vi "DAQ IV.vi"() -> ()   [LabVIEW 2024]
uses:
  global.vi
panel:
  in  "base path":path=path "C:/Users/gyue/Desktop/20211027"
  out "Voltage Applied":dbl=-2.0
  in  "Tab Control":enum32{"Curve Control", "Setup"}(tab)
  in  "Voltage Offset":dbl caption="Delay Time (s)" format="%#_4f"
  in  "End Current uA":dbl=2.0
  in  "Start Current uA":dbl=-2.0
  in  "Step uA":dbl=0.05
  in  "Delay Time s":dbl caption="Delay Time (s)"
  in  "True is round":bool=TRUE
  in  "Current scale":dbl=1.0 caption="Delay Time (s)" format="%#_5f"
  in  "Voltage scale":dbl=0.0001 caption="Delay Time (s)" format="%#_4f"
  in  "Wire Resistance":dbl caption="Delay Time (s)" format="%#_6f"
  in  "AO channel":tag="Dev1/ao0"
  in  "AI channel":tag="Dev1/ai1"
  in  "samples per read":i32=1000
  in  "device in":tag="Dev1"
  in  "stop 2":bool
  in  "stop":bool
  out "Cursor measured \nResistance Ohm":dbl=20.21557814005861
  in  "error in":T1
  out "Current Applied":dbl=-2.0
  out "Voltage":dbl=-2.7920312698574086e-05 format="%^#_4g"
  out "IV curve":cluster{"Y":dbl[], "Y":dbl[]}[](graph)=[{"Y"=[-2.0, -1.95, -1.9, -1.85, -1.8, -1.75, -1.7, -1.65, -1.6, -1.55, -1.5, -1.45, -1.4, -1.35, -1.2999999999999998, -1.25, -1.2, -1.15, -1.1, -1.0499999999999998, -1.0, -0.95, -0.8999999999999999, -0.8499999999999999, -0.7999999999999998, -0.75, -0.7, -0.6499999999999999, -0.5999999999999999, -0.5499999999999998, -0.5, -0.44999999999999996, -0.3999999999999999, -0.34999999999999987, -0.2999999999999998, -0.25, -0.19999999999999996, -0.1499999999999999, -0.09999999999999987, -0.04999999999999982, 0.0, 0.050000000000000266, 0.10000000000000009, 0.1499999999999999, 0.20000000000000018, 0.25, 0.30000000000000027, 0.3500000000000001, 0.40000000000000036, 0.4500000000000002, 0.5, 0.5500000000000003, 0.6000000000000001, 0.6500000000000004, 0.7000000000000002, 0.75, 0.8000000000000003, 0.8500000000000001, 0.9000000000000004, 0.9500000000000002, 1.0, 1.0500000000000003, 1.1, 1.1500000000000004, 1.2000000000000002, 1.25, 1.3000000000000003, 1.35, 1.4000000000000004, 1.4500000000000002, 1.5, 1.5500000000000003, 1.6, 1.6500000000000004, 1.7000000000000002, 1.75, 1.8000000000000003, 1.85, 1.9000000000000004, 1.9500000000000002, 2.0, 1.9500000000000002, 1.8999999999999995, 1.8499999999999996, 1.7999999999999998, 1.75, 1.7000000000000002, 1.6499999999999995, 1.5999999999999996, 1.5499999999999998, 1.5, 1.4500000000000002, 1.3999999999999995, 1.3499999999999996, 1.2999999999999998, 1.25, 1.1999999999999993, 1.1499999999999995, 1.0999999999999996, 1.0499999999999998, 1.0, 0.9499999999999993, 0.8999999999999995, 0.8499999999999996, 0.7999999999999998, 0.75, 0.6999999999999993, 0.6499999999999995, 0.5999999999999996, 0.5499999999999998, 0.5, 0.4499999999999993, 0.39999999999999947, 0.34999999999999964, 0.2999999999999998, 0.25, 0.1999999999999993, 0.14999999999999947, 0.09999999999999964, 0.04999999999999982, 0.0, -0.05000000000000071, -0.10000000000000053, -0.15000000000000036, -0.20000000000000018, -0.25, -0.3000000000000007, -0.35000000000000053, -0.40000000000000036, -0.4500000000000002, -0.5, -0.5500000000000007, -0.6000000000000005, -0.6500000000000004, -0.7000000000000002, -0.75, -0.8000000000000007, -0.8500000000000005, -0.9000000000000004, -0.9500000000000002, -1.0, -1.0500000000000007, -1.1000000000000005, -1.1500000000000004, -1.2000000000000002, -1.25, -1.3000000000000007, -1.3500000000000005, -1.4000000000000004, -1.4500000000000002, -1.5, -1.5500000000000007, -1.6000000000000005, -1.6500000000000004, -1.7000000000000002, -1.75, -1.8000000000000007, -1.8500000000000005, -1.9000000000000004, -1.9500000000000002, -2.0], "Y"=[-2.7806350133557928e-05, -2.6315904493930977e-05, -2.5254383611053963e-05, -2.4587024225926712e-05, -2.3728933259964108e-05, -2.3027212849366328e-05, -2.2141665286220923e-05, -2.1379318299329873e-05, -2.0517557855817245e-05, -1.9756804202124692e-05, -1.9050480919686794e-05, -1.81145104290271e-05, -1.7234965967061796e-05, -1.6725007221815502e-05, -1.0688692788176573e-05, 3.3718837287303505e-06, 4.087509465991185e-06, 3.849268038827346e-06, 3.8973411331160935e-06, 3.929738627589131e-06, 3.987307418668881e-06, 3.8987896840092175e-06, 4.008583844587979e-06, 4.122916555804554e-06, 4.290826659842316e-06, 4.170265544331957e-06, 3.399726578537852e-06, 3.559042433568257e-06, 3.772498938509106e-06, 4.161542498920955e-06, 4.0600206975398566e-06, 4.178473496306829e-06, 4.0578962701376445e-06, 4.099531771424895e-06, 3.892545061847544e-06, 3.903617849968508e-06, 4.016019312818286e-06, 3.840110421224071e-06, 3.3714008916531e-06, 3.9287891200741636e-06, 3.750868427469185e-06, 3.6483809777301958e-06, 3.777761713750314e-06, 3.7623757445817637e-06, 3.89915976555755e-06, 3.812557244971531e-06, 3.8237909354108325e-06, 3.0537187878291632e-06, 2.8061587728981296e-06, 2.880706824887942e-06, 3.004921328843233e-06, 2.572391451368744e-06, 3.1258687647810383e-06, 3.879508832811618e-06, 3.7155578662921936e-06, 3.7816404098090527e-06, 3.5493698315194495e-06, 3.7760074725172656e-06, 3.581075289327683e-06, 3.3063162503447812e-06, 3.5696645300099503e-06, 3.7209493952618246e-06, 3.81675777625176e-06, 3.6615298851288586e-06, 4.274652035225237e-06, 9.718912254674585e-06, 2.1385905901929005e-05, 2.3813674250206032e-05, 2.5083920209590195e-05, 2.5892103419971726e-05, 2.697567371138931e-05, 2.7447795105974072e-05, 2.810384056996338e-05, 2.8688830224305425e-05, 2.9239523490006232e-05, 3.01782946916214e-05, 3.146896424793762e-05, 3.252795847887403e-05, 3.29581065594398e-05, 3.372240119791277e-05, 3.467039449610606e-05, 3.3939575506465646e-05, 3.337568526030103e-05, 3.248360304918371e-05, 3.145761769628095e-05, 3.097460047538676e-05, 2.9951479862093785e-05, 2.9193236717165506e-05, 2.8354522853339044e-05, 2.7677925226732942e-05, 2.7024471044186455e-05, 2.5768387841127474e-05, 2.4886493374053423e-05, 2.3967260631142617e-05, 2.3511168829961115e-05, 2.2559779971435673e-05, 1.88101197817795e-05, 9.342148473014151e-06, 3.659019139000812e-06, 3.404200762398993e-06, 3.7212070033125773e-06, 3.847417184515833e-06, 3.1033530512071833e-06, 3.291750999617621e-06, 3.5202394876931186e-06, 3.64696468430102e-06, 3.2951951619687253e-06, 3.464650381635116e-06, 3.1600366595496455e-06, 3.1183367181168565e-06, 3.0507091730994633e-06, 3.069571526872606e-06, 3.0994905135569186e-06, 3.3632894776910013e-06, 2.7063590900957317e-06, 2.8254718035328737e-06, 3.0811270886767434e-06, 3.2866169950753825e-06, 2.647937295989086e-06, 3.1799772505856613e-06, 3.585517308438334e-06, 3.796302150748738e-06, 3.8432326414386725e-06, 3.6510364983768703e-06, 3.608612360626172e-06, 3.379946914075492e-06, 3.5525886590308885e-06, 3.257325658305754e-06, 3.4552192015453656e-06, 3.591761818003331e-06, 3.284186774791432e-06, 2.973763107466172e-06, 3.0107796037187713e-06, 3.0837826258433704e-06, 3.1480625725063823e-06, 3.042806940510062e-06, 2.9947176880653673e-06, 2.8626009213047656e-06, 3.112253159167387e-06, 3.0546039377523047e-06, 3.4385778357676433e-06, 3.5091184247574418e-06, 3.530137376554258e-06, 3.551687436492003e-06, 2.5253322629098626e-06, -8.498474149084183e-06, -1.624664126215314e-05, -1.684927003511216e-05, -1.7760358996592866e-05, -1.8559078711569726e-05, -1.9051945488442992e-05, -2.042290825163416e-05, -2.1236804747515748e-05, -2.179601154109642e-05, -2.30205981708698e-05, -2.3247622035734454e-05, -2.4922554733722028e-05, -2.5875520672008874e-05, -2.652343836305606e-05, -2.7159736078887955e-05, -2.7920312698574086e-05]}]
  out "error out":errorcluster
  # "I uA * scale= Voutput\nV Read * scale=actual V"
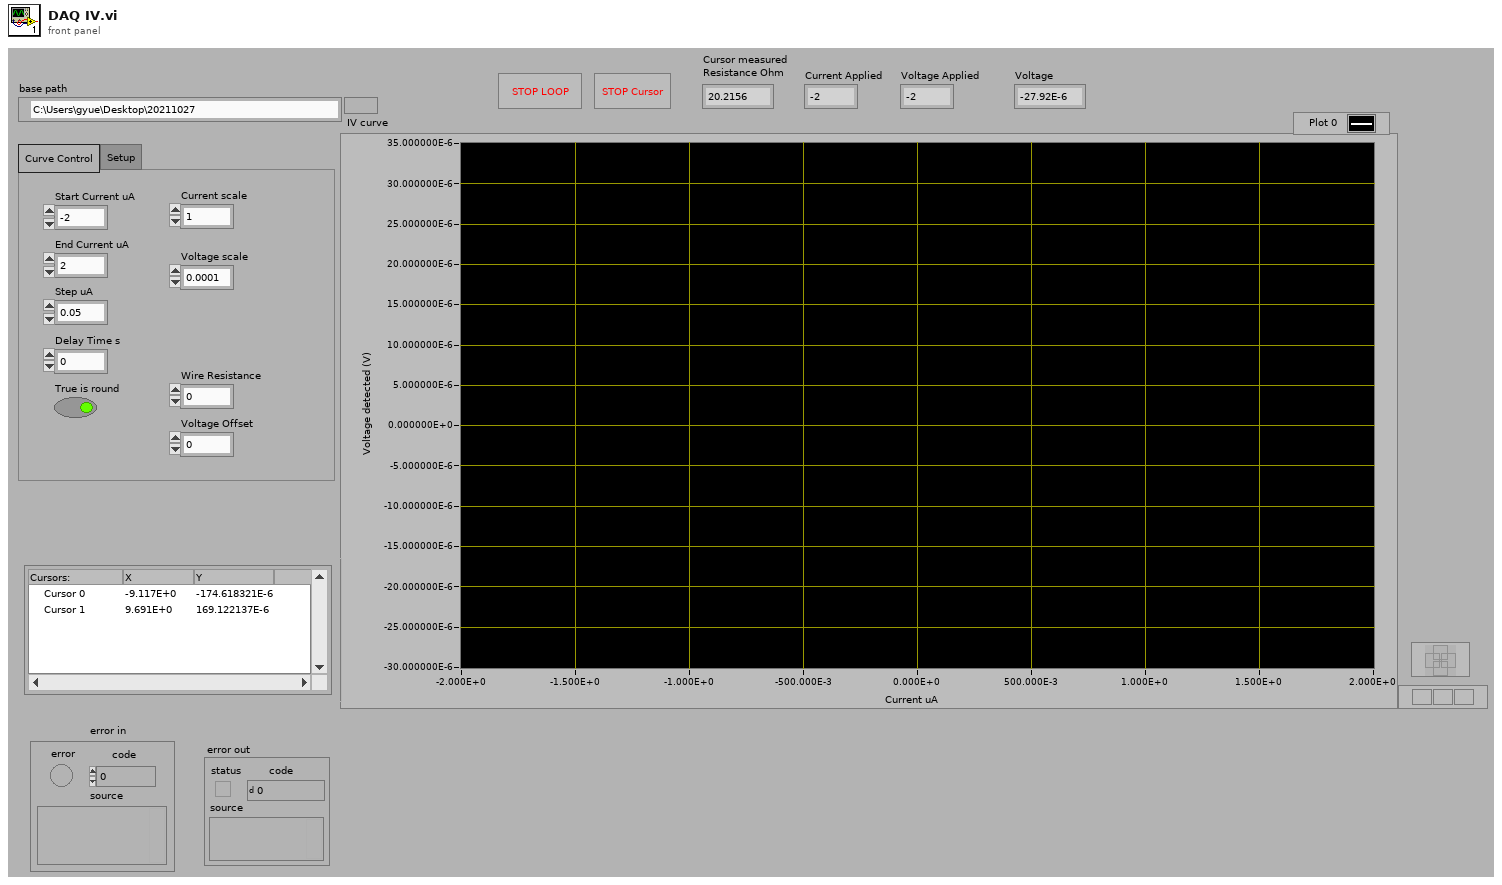
[diagram p1: front panel]
types:
  T1 = cluster{"error":bool, "code":i32, "source":string}
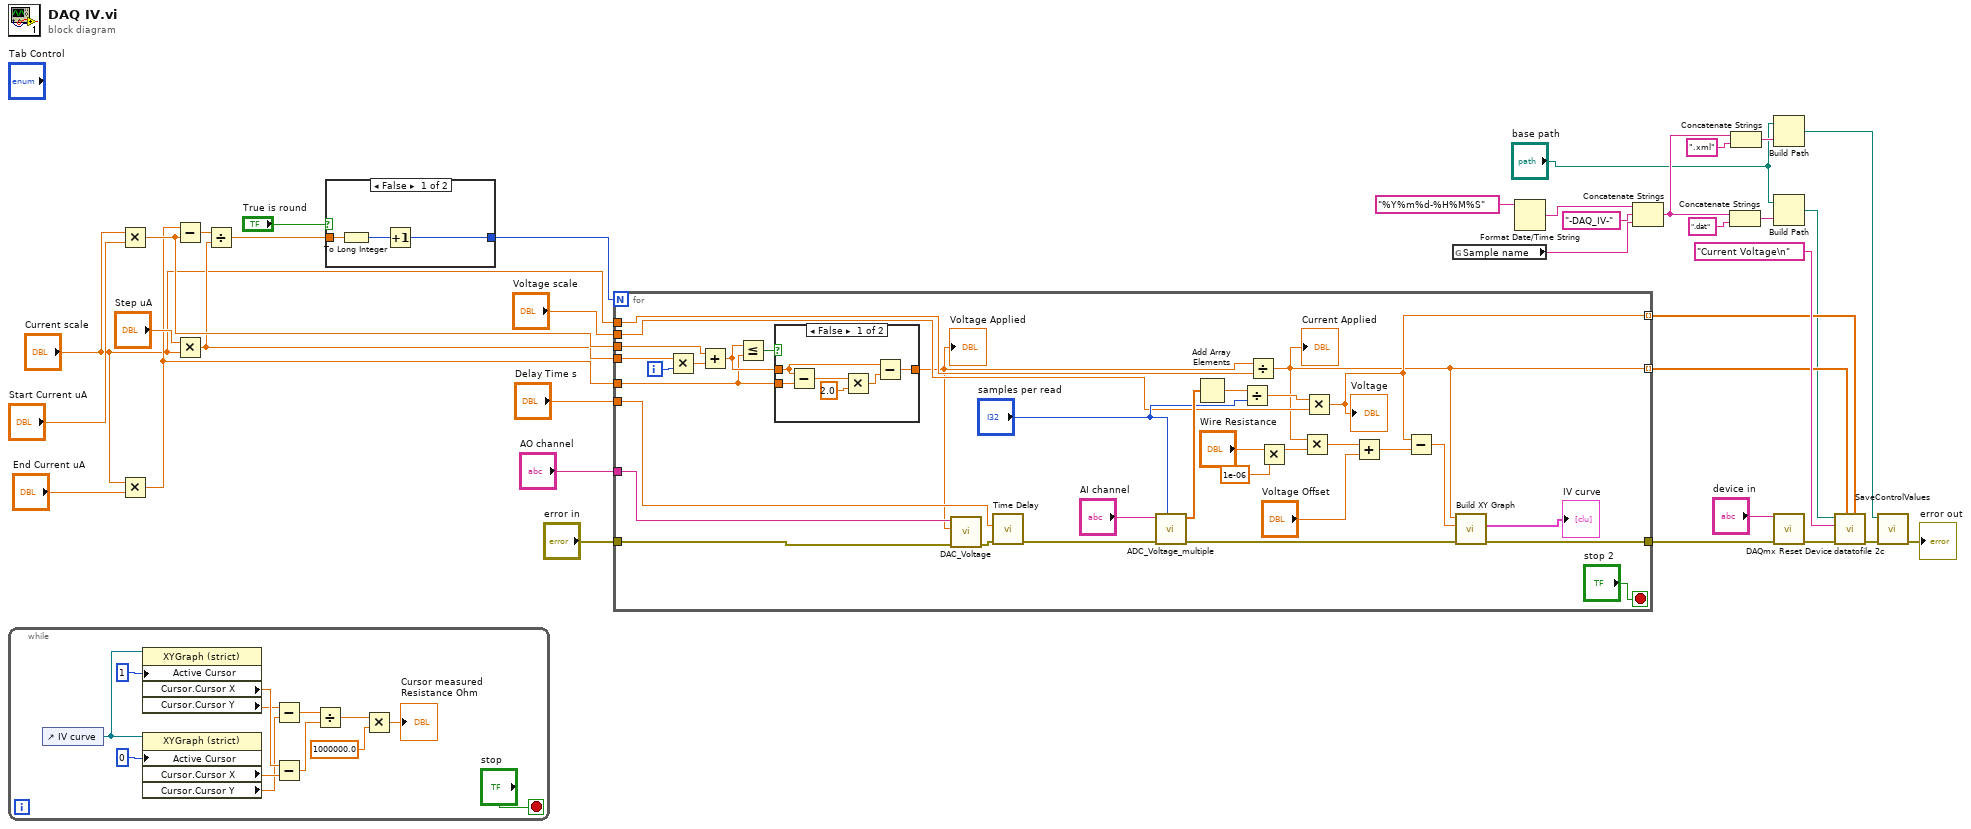
[diagram p0: block diagram]
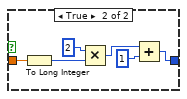
[diagram p2: hidden frame]
diagram:
  n1 = while {
    stop <- "stop" stop-if-true
    n2 = control-ref of="IV curve"() -> (w36:refnum<vi>)
    n3 = property class="XYGraph (strict)"(reference=w36, "Active Cursor"=u32 1) -> ("Cursor.Cursor X"=w41:dbl, "Cursor.Cursor Y"=w39:dbl)  [unwired: 1 in, 2 out]
    n4 = property class="XYGraph (strict)"(reference=w36, "Active Cursor"=u32 0) -> ("Cursor.Cursor X"=w42:dbl, "Cursor.Cursor Y"=w40:dbl)  [unwired: 1 in, 2 out]
    n5 = Subtract(x=w39, y=w40) -> (x-y=w43:dbl)
    n6 = Subtract(x=w41, y=w42) -> (x-y=w44:dbl)
    n7 = Divide(x=w43, y=w44) -> (x/y=w45:dbl)
    n8 = Multiply(x=w45, y=1000000.0) -> (x*y=→"Cursor measured \nResistance Ohm":dbl)
  }
  n9 = Multiply(x="Current scale", y="Start Current uA") -> (x*y=w6:dbl)
  n10 = Multiply(x="Current scale", y="End Current uA") -> (x*y=w5:dbl)
  n11 = Subtract(x=w5, y=w6) -> (x-y=w35:dbl)
  n12 = Multiply(x="Step uA", y="Current scale") -> (x*y=w4:dbl)
  n13 = Divide(x=w35, y=w4) -> (x/y=w34:dbl)
  n14 = case shown="False" "True is round" {
    tunnel: w34 -> [w51 w57]
    tunnel: [w49 w55] -> w33
    frame False {
      n15 = To Long Integer(number=w51) -> (32bit integer=w50:i32)
      n16 = Increment(x=w50) -> (x+1=w49:i32)
    }
    frame True {
      n17 = To Long Integer(number=w57) -> (32bit integer=w53:i32)
      n18 = Multiply(x=2, y=w53) -> (x*y=w54:i32)
      n19 = Add(x=w54, y=1) -> (x+y=w55:i32)
    }
  }
  n20 = for {
    N: w33 -> [_]
    tunnel: w6 -> [w87]
    tunnel: w4 -> [w89]
    tunnel: w5 -> [w84]
    tunnel: [w82] -> w9
    tunnel: [w64] -> w28 mode=indexing
    tunnel: [w66] -> w27 mode=indexing
    tunnel: "error in" -> [w79]
    tunnel: "Delay Time s" -> [w81]
    tunnel: "AO channel" -> [w75]
    tunnel: "Voltage scale" -> [w69]
    tunnel: "Current scale" -> [w68]
    i -> [w90]
    stop <- "stop 2" stop-if-true
    n21 = Multiply(x=w89, y=w90) -> (x*y=w88:dbl)
    n22 = Add(x=w87, y=w88) -> (x+y=w85:dbl)
    n23 = Less Or Equal?(x=w85, y=w84) -> (x <= y?=w86:bool)
    n24 = case shown="False" w86 {
      tunnel: [w94 w97] -> w67
      tunnel: w85 -> [w95 w97]
      tunnel: w84 -> [w96 _]
      frame False {
        n25 = Subtract(x=w95, y=w96) -> (x-y=w93:dbl)
        n26 = Multiply(x=w93, y=2.0) -> (x*y=w91:dbl)
        n27 = Subtract(x=w95, y=w91) -> (x-y=w94:dbl)
      }
      frame True {
      }
    }
    "Voltage Applied" <- w67
    n28 = call "DAC_Voltage.vi"("error in"=w79, "Voltage"=w67, "Physical Channel(s)"=w75) -> ("error out"=w78:errorcluster)  [unwired: 8 in]
    n29 = call "Time Delay"("error in (no error)"=w78, "Delay Time (s)"=w81) -> ("error out"=w77:errorcluster)  [unwired: 9 in]
    n30 = call "ADC_Voltage_multiple.vi"("samples per channel"="samples per read", "error in"=w77, "physical channels"="AI channel") -> ("error out"=w76:errorcluster, "data"=w73:dbl[])  [unwired: 7 in]
    n31 = Add Array Elements(numeric array=w73) -> (sum=w72:dbl)
    n32 = Divide(x=w72, y="samples per read") -> (x/y=w70:dbl)
    n33 = Divide(x=w67, y=w68) -> (x/y=w64:dbl)
    "Current Applied" <- w64
    n34 = Multiply(x="Wire Resistance", y=1e-06) -> (x*y=w59:dbl)
    n35 = Multiply(x=w64, y=w59) -> (x*y=w63:dbl)
    n36 = Multiply(x=w70, y=w69) -> (x*y=w66:dbl)
    "Voltage" <- w66
    n37 = Add(x=w63, y="Voltage Offset") -> (x+y=w61:dbl)
    n38 = Subtract(x=w66, y=w61) -> (x-y=w60:dbl)
    n39 = call "Build XY Graph"("error in (no error)"=w76, "Y Input"=w60, "X Input"=w64) -> ("error out"=w82:errorcluster, "XY Graph"=→"IV curve":cluster{"Y":dbl[], "Y":dbl[]}[])  [unwired: 7 in]
  }
  n40 = global read "global.vi" "Sample name"() -> (w19:string)
  n41 = Format Date/Time String(time format string (%c)="%Y%m%d-%H%M%S") -> (date/time string=w21:string)  [unwired: 2 in]
  n42 = Concatenate Strings(w21, "-DAQ_IV-" ("string"), w19) -> (w16:string)
  n43 = Concatenate Strings(w16, ".dat" ("string")) -> (w17:string)
  n44 = Concatenate Strings(w16, ".xml" ("string")) -> (w14:string)
  n45 = Build Path(base path="base path", name or relative path=w14) -> (appended path=w13:path)
  n46 = Build Path(base path="base path", name or relative path=w17) -> (appended path=w23:path)
  n47 = call <vilib>:"DAQmx Reset Device.vi"("device in"="device in", "error in"=w9) -> ("error out"=w8:errorcluster)  [unwired: 13 in]
  n48 = call "datatofile 2c.vi"("A2"=w27, "A1"=w28, "error in"=w8, "title"="Current Voltage\n", "file path (dialog if empty)"=w23) -> ("error out"=w12:errorcluster)  [unwired: 6 in]
  n49 = call "SaveControlValues.vi"("XML File Path"=w13, "error in (no error)"=w12) -> ("error out"=→"error out":errorcluster)  [unwired: 8 in]
